vi "Visit Me.vi"(8 "error in (no error)":errorcluster, 10 "Visitor In":refnum<class "LVTypeVisitor.lvclass">, 11 "LVAnalogWaveformType in":refnum<class "LVAnalogWaveformType.lvclass">) -> (0 "error out":errorcluster, 2 "Visitor Out":refnum<class "LVTypeVisitor.lvclass">, 3 "LVAnalogWaveformType out":refnum<class "LVAnalogWaveformType.lvclass">)   [LabVIEW 2020, in "LVDataTypes.lvlib" / "LVAnalogWaveformType.lvclass"]
uses:
  <vilib>/AppBuilder/Engine/WebServiceDescription/LVDataTypes/LVAnalogWaveformType/LVAnalogWaveformType.lvclass
  <vilib>/AppBuilder/Engine/WebServiceDescription/LVDataTypes/LVTypeVisitor/LVTypeVisitor.lvclass
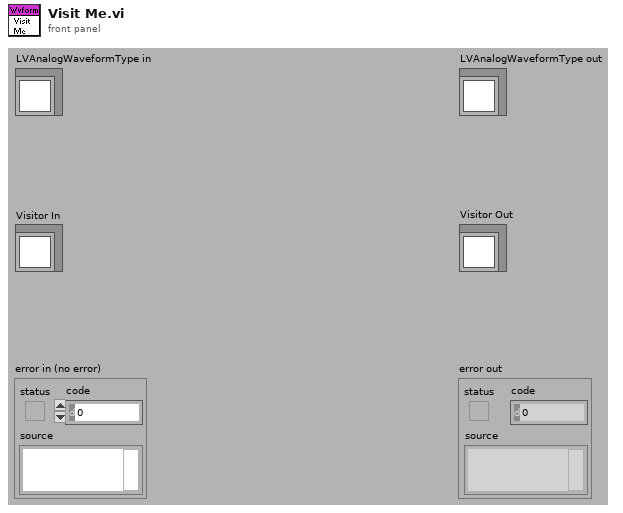
[diagram p1: front panel]
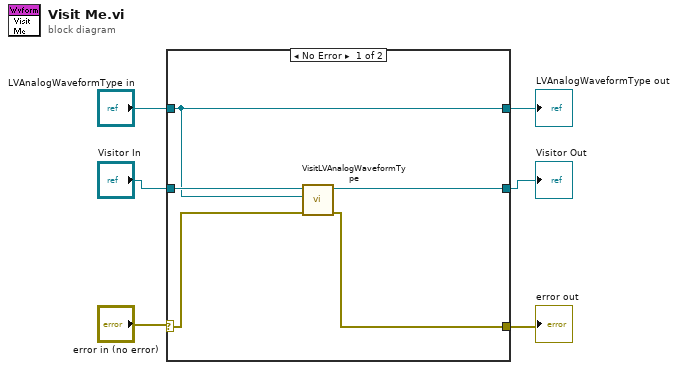
[diagram p0: block diagram]
diagram:
  n1 = case shown="No Error" "error in (no error)" {
    selector: "error in (no error)" -> [w9 w14]
    tunnel: [w8 w14] -> w5
    tunnel: [w7 w13] -> w3
    tunnel: "Visitor In" -> [w11 w13]
    tunnel: "LVAnalogWaveformType in" -> [w10 w12]
    tunnel: [w10 w12] -> w1
    frame No Error {
      n2 = call-dynamic "VisitLVAnalogWaveformType.vi"("error in (no error)"=w9, "LVAnalogWaveformType"=w10, "LVTypeVisitor in"=w11) -> ("error out"=w8:errorcluster, "LVTypeVisitor out"=w7:refnum<class "LVTypeVisitor.lvclass">)  [unwired: 7 out]
    }
    frame Error {
    }
  }
  "error out" <- w5
  "LVAnalogWaveformType out" <- w1
  "Visitor Out" <- w3
